vi "Configure Reference Waveform.vi"   [LabVIEW 2010, in "Agilent 2000 3000 X-Series.lvlib"]
doc: "Configures reference waveform."
uses:
  <instrlib>/Agilent 2000 3000 X-Series/Agilent 2000 3000 X-Series.lvlib
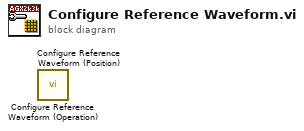
[diagram p0: block diagram]
diagram:
  n1 = call <instrlib>:"Configure Reference Waveform (Operation).vi"() -> ()  [unwired: 10 in, 2 out]
  n2 = call <instrlib>:"Configure Reference Waveform (Position).vi"() -> ()  [unwired: 10 in, 2 out]
